vi "Connecting.vi"(11 "System Data":T1={"System"={"Active"=FALSE, "Exit"=FALSE, "Command wait"="", "Status_Time"=0, "Time_GPS"=0}, "Stepper Motor"={"Connection Reference"="", "Valid Connection"=FALSE, "Speed"=15}, "Camera Data"={"Image path"=path "", "Filenames"=[], "Filenames queue"=[]}, "Core"={"Close Panel on Exit?"=FALSE, "Current VI Reference"=refnum}} {"Stepper Motor"."Speed" scale=0.0..30.0}) -> (3 "System Data out":T1={"System"={"Active"=FALSE, "Exit"=FALSE, "Command wait"="", "Status_Time"=0, "Time_GPS"=0}, "Stepper Motor"={"Connection Reference"="", "Valid Connection"=FALSE, "Speed"=15}, "Camera Data"={"Image path"=path "", "Filenames"=[], "Filenames queue"=[]}, "Core"={"Close Panel on Exit?"=FALSE, "Current VI Reference"=refnum}} {"Stepper Motor"."Speed" scale=0.0..30.0})   [LabVIEW 2019]
uses:
  System Data.ctl
  Stepper Data.ctl
  Camera Data.ctl
  ce23ff2a-da51-4feb-a7c7-56550c1584c2.vi
  <extravilib>/ChannelInstances/Tag-u16[Search,Search error,Connect,Connection complete,Connect Error]/Read With Abort.vi
  <extravilib>/ChannelInstances/Tag-bool/Write With Abort.vi
  <extravilib>/ChannelInstances/Tag-u16[Search,Search error,Connect,Connection complete,Connect Error]/Write With Abort.vi
  <extravilib>/ChannelInstances/Tag-bool/Instantiate.vi
  <extravilib>/ChannelInstances/Tag-u16[Search,Search error,Connect,Connection complete,Connect Error]/Instantiate.vi
  <extravilib>/ChannelInstances/Tag-u16[Search,Search error,Connect,Connection complete,Connect Error]/Endpoint.vi
  <extravilib>/ChannelInstances/Tag-u16[Search,Search error,Connect,Connection complete,Connect Error]/EndpointRead.vi
  <extravilib>/ChannelInstances/Tag-bool/Endpoint.vi
  <extravilib>/ChannelInstances/Tag-u16[Search,Search error,Connect,Connection complete,Connect Error].lvlib
  <extravilib>/ChannelInstances/Tag-bool.lvlib
panel:
  out "Connect":dbl(ring)=14.0
  out "Connect":string
  in  "OK":bool
  out "Search":dbl(ring)
  out "Search":string="Searching for system"
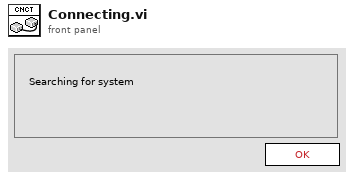
[diagram p1: front panel]
types:
  T1 = typedef "System Data.ctl" = cluster{"System":cluster{"Active":bool, "Exit":bool, "Command wait":string, "Status_Time":i32, "Time_GPS":i32}, "Stepper Motor":T2, "Camera Data":T3, "Core":cluster{"Close Panel on Exit?":bool, "Current VI Reference":refnum<vi>}}
  T2 = typedef "Stepper Data.ctl" = cluster{"Connection Reference":refnum<visa-resource-name>, "Valid Connection":bool, "Speed":i32}
  T3 = typedef "Camera Data.ctl" = cluster{"Image path":path, "Filenames":string[], "Filenames queue":string[]}
  T4 = enum16{"Search", "Search error", "Connect", "Connection complete", "Connect Error"}
  T5 = typedef "Tag-u16[Search,Search error,Connect,Connection complete,Connect Error].lvlib/))Channel.ctl" = refnum<queue>
  T6 = enum8{"Enabled", "Disabled", "Disabled and Grayed Out"}
  T7 = typedef "Tag-bool.lvlib/))Channel.ctl" = refnum<queue>
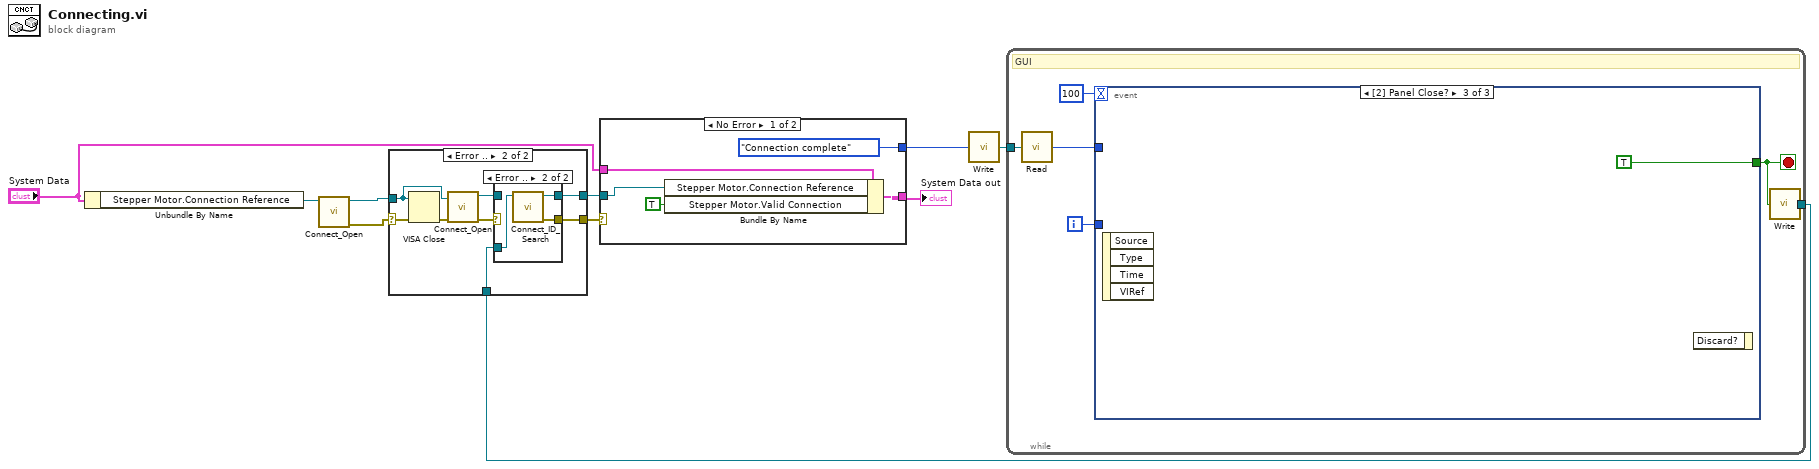
[diagram p0: block diagram]
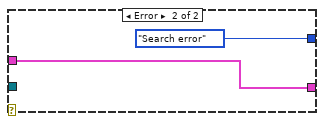
[diagram p4: hidden frame]
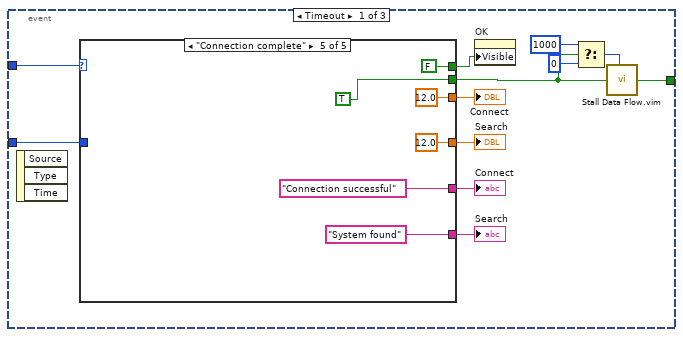
[diagram p5: hidden frame]
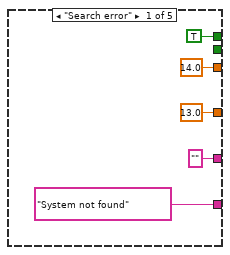
[diagram p6: hidden frame]
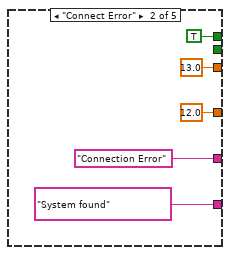
[diagram p7: hidden frame]
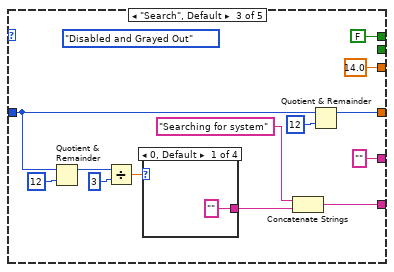
[diagram p8: hidden frame]
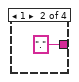
[diagram p9: hidden frame]
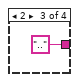
[diagram p10: hidden frame]
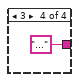
[diagram p11: hidden frame]
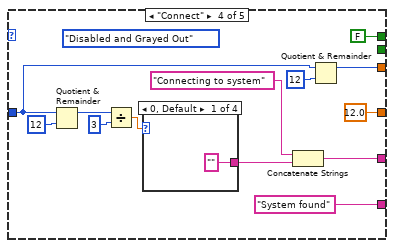
[diagram p12: hidden frame]
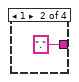
[diagram p13: hidden frame]
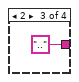
[diagram p14: hidden frame]
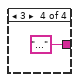
[diagram p15: hidden frame]
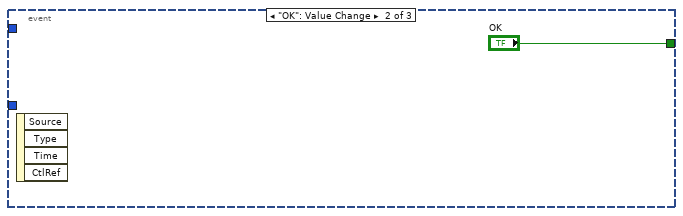
[diagram p16: hidden frame]
diagram:
  n1 = Unbundle By Name("System Data") -> ("Stepper Motor.Connection Reference"=w7:refnum<visa-resource-name>)
  n2 = call "Connect_Open.vi"("VISA Refnum in"=w7) -> ("error out"=w1:errorcluster, "VISA Refnum out"=w2:refnum<visa-resource-name>)  [unwired: 9 in]
  n3 = case shown="Error .." w1 {
    selector: w1 -> [w12 w17]
    tunnel: [w12 w20] -> w8
    tunnel: [w11 w19] -> w6
    tunnel: w4 -> [_ w18]
    tunnel: w2 -> [w11 w16]
    frame No Error {
    }
    frame Error {
      n4 = VISA Close(VISA resource name=w16, error in (no error)=w17) -> (error out=w15:errorcluster)
      n5 = call "Connect_Open.vi"("error in (no error)"=w15, "VISA Refnum in"=w16) -> ("error out"=w14:errorcluster, "VISA Refnum out"=w13:refnum<visa-resource-name>)  [unwired: 8 in]
      n6 = case shown="Error .." w14 {
        selector: w14 -> [w22 _]
        tunnel: [w22 w25] -> w20
        tunnel: [w21 w24] -> w19
        tunnel: w18 -> [_ w23]
        tunnel: w13 -> [w21 _]
        frame No Error {
        }
        frame Error {
          n7 = call "Connect_ID_Search.vi"("channel"=w23) -> ("error out"=w25:errorcluster, "Arduino Ref"=w24:refnum<visa-resource-name>)  [unwired: 9 in]
        }
      }
    }
  }
  n8 = case shown="No Error" w8 {
    tunnel: [T4."Connection complete" ("element") T4."Search error" ("element")] -> w9
    tunnel: "System Data" -> [w29 w31]
    tunnel: w6 -> [w28 _]
    tunnel: [w27 w31] -> w5
    frame No Error {
      n9 = Bundle By Name(cluster=w29, "Stepper Motor.Connection Reference"=w28, "Stepper Motor.Valid Connection"=TRUE) -> (w27:T1)
    }
    frame Error {
    }
  }
  "System Data out" <- w5
  n10 = call <extravilib>:"Write.vi"("element"=w9) -> ("channel"=w10:T5)  [unwired: 1 out]
  n11 = while {
    tunnel: w10 -> [w36]
    tunnel: [w33] -> w4
    i -> [w37]
    stop <- w34 stop-if-true
    # "GUI"
    n12 = call <extravilib>:"Read.vi"("channel"=w36) -> ("element"=w35:T4)  [unwired: 1 in, 1 out]
    n13 = event shown="[2] Panel Close?" {
      selector: _ -> [_ _ _]
      dyn-events: _ -> [_ _ _]
      timeout: u32 100 ("milliseconds to wait") -> [_ _ _]
      tunnel: w37 -> [w49 _ _]
      tunnel: [w43 "OK" TRUE ("Stop")] -> w34
      tunnel: w35 -> [w45 _ _]
      event Timeout {
        n14 = event-data() -> ()  [unwired: 1 in, 3 out]
        n15 = case shown="\"Connection complete\"" w45 {
          tunnel: ["System not found" ("String") "System found" ("String") w72 "System found" ("string") "System found" ("string")] -> w50
          tunnel: w49 -> [_ _ w71 w89 _]
          tunnel: [13.0 12.0 w68 12.0 ("Pict Ring 2") 12.0 ("Pict Ring 2")] -> w48
          tunnel: ["" ("string") "Connection Error" ("string") "" ("string") w82 "Connection successful" ("string")] -> w47
          tunnel: [14.0 ("Pict Ring 2") 13.0 ("Pict Ring 2") 14.0 ("Pict Ring 2") w81 12.0 ("Pict Ring 2")] -> w46
          tunnel: [TRUE ("Visible") TRUE ("Visible") FALSE ("Visible") FALSE ("Visible") FALSE ("Visible")] -> w44
          tunnel: [_ _ _ _ TRUE ("Visible")] -> w42
          frame "Search error" {
          }
          frame "Connect Error" {
          }
          frame "Search", Default {
            (unwired) T6."Disabled and Grayed Out" ("Disabled")
            n16 = Quotient & Remainder(x=w71, y=12) -> (x-y*floor(x/y)=w69:i32)  [unwired: 1 out]
            n17 = Divide(x=w69, y=3 ("x")) -> (x/y=w67:dbl)
            n18 = case shown="0, Default" w67 {
              tunnel: ["" "." ".." "..."] -> w64
              frame 0, Default {
              }
              frame 1 {
              }
              frame 2 {
              }
              frame 3 {
              }
            }
            n19 = Concatenate Strings("Searching for system" ("string"), w64) -> (w72:string)
            n20 = Quotient & Remainder(x=w71, y=12) -> (x-y*floor(x/y)=w68:i32)  [unwired: 1 out]
          }
          frame "Connect" {
            (unwired) T6."Disabled and Grayed Out" ("Disabled")
            n21 = Quotient & Remainder(x=w89, y=12) -> (x-y*floor(x/y)=w87:i32)  [unwired: 1 out]
            n22 = Divide(x=w87, y=3 ("x")) -> (x/y=w86:dbl)
            n23 = case shown="0, Default" w86 {
              tunnel: ["" "." ".." "..."] -> w83
              frame 0, Default {
              }
              frame 1 {
              }
              frame 2 {
              }
              frame 3 {
              }
            }
            n24 = Concatenate Strings("Connecting to system" ("string"), w83) -> (w82:string)
            n25 = Quotient & Remainder(x=w89, y=12) -> (x-y*floor(x/y)=w81:i32)  [unwired: 1 out]
          }
          frame "Connection complete" {
          }
        }
        "Search" <- w48
        "Search" <- w50
        "Connect" <- w47
        "Connect" <- w46
        n26 = property on="OK" class="Bool"("Visible"=w44) -> ()  [unwired: 2 in, 2 out]
        n27 = Select(t=1000, s=w42, f=0) -> (s? t:f=w39:i32)
        n28 = call "Stall Data Flow.vim"("value in"=w42, "milliseconds to wait"=w39) -> ("value out"=w43:bool)  [unwired: 1 out]
      }
      event "OK": Value Change {
        n29 = event-data() -> ()  [unwired: 1 in, 4 out]
      }
      event Panel Close? {
        n30 = event-data() -> ()  [unwired: 1 in, 4 out]
        n31 = event-data() -> ()  [unwired: 2 in, 1 out]
      }
    }
    n32 = call <extravilib>:"Write.vi"("element"=w34) -> ("channel"=w33:T7)  [unwired: 1 out]
  }
